vi "Configure Average.vi"(7 "Average On (F)":bool, 8 "error in (no error)":errorcluster, 10 "Average":u32, 11 "SA-ESA in":refnum<class "SA-ESA.lvclass">) -> (0 "error out":errorcluster, 3 "SA-ESA out":refnum<class "SA-ESA.lvclass">)   [LabVIEW 2020, in "SA-ESA.lvclass"]
uses:
  SA-ESA.lvclass
  C:/Sandbox/Git_Sandbox/WiSpry Test Framework source code (LV20)/WiSpry Test Framework/Instruments/Instrument.lvclass
  C:/Sandbox/Git_Sandbox/WiSpry Test Framework source code (LV20)/WiSpry Test Framework/Instruments/Spectrum Analyzer/Spectrum Analyzer.lvclass
  Spectrum Analyzer.lvclass/Spectrum Analyzer.ctl
  Instrument.lvclass/Instrument.ctl
  Instrument.lvclass
  Spectrum Analyzer.lvclass
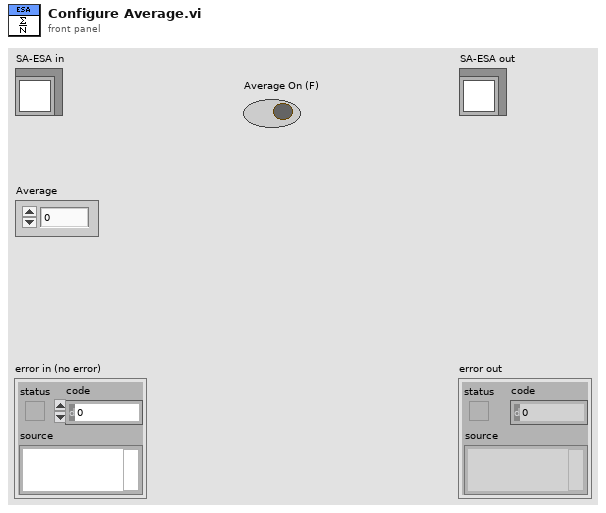
[diagram p1: front panel]
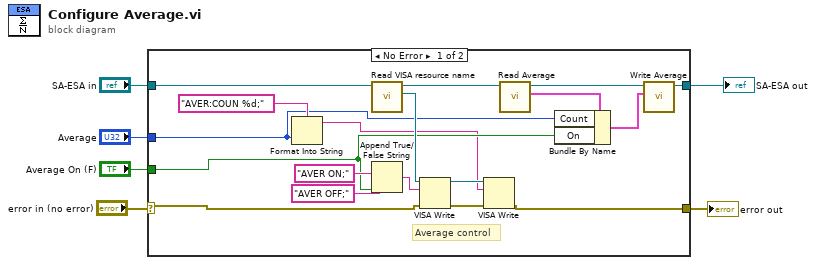
[diagram p0: block diagram]
diagram:
  n1 = case shown="No Error" "error in (no error)" {
    selector: "error in (no error)" -> [w18 w25]
    tunnel: "SA-ESA in" -> [w20 w26]
    tunnel: "Average" -> [w15 _]
    tunnel: "Average On (F)" -> [w14 _]
    tunnel: [w11 w26] -> w2
    tunnel: [w7 w25] -> w1
    frame No Error {
      # "Average control"
      n2 = Format Into String(format string="AVER:COUN %d;", w15) -> (resulting string=w8:string)  [unwired: 2 in, 1 out]
      n3 = call "Read VISA resource name.vi"("Instrument in"=w20) -> ("VISA resource name"=w19:refnum<visa-resource-name>, "Instrument out"=w17:refnum<class "SA-ESA.lvclass">)  [unwired: 9 in]
      n4 = Append True/False String(1:w14, 2:"AVER OFF;" ("false string"), 3:"AVER ON;" ("true string")) -> (0:w21:string)  [unwired: 1 in]
      n5 = VISA Write(VISA resource name=w19, write buffer=w21, error in (no error)=w18) -> (VISA resource name out=w9:refnum<visa-resource-name>, error out=w10:errorcluster)  [unwired: 1 out]
      n6 = VISA Write(VISA resource name=w9, write buffer=w8, error in (no error)=w10) -> (error out=w7:errorcluster)  [unwired: 2 out]
      n7 = call "Read Average.vi"("Spectrum Analyzer in"=w17) -> ("Average"=w16:cluster{"Count":u32, "On":bool}, "Spectrum Analyzer out"=w13:refnum<class "SA-ESA.lvclass">)  [unwired: 9 in]
      n8 = Bundle By Name(cluster=w16, "Count"=w15, "On"=w14) -> (w12:cluster{"Count":u32, "On":bool})
      n9 = call "Write Average.vi"("Average"=w12, "Spectrum Analyzer in"=w13) -> ("Spectrum Analyzer out"=w11:refnum<class "SA-ESA.lvclass">)  [unwired: 9 in]
    }
    frame Error {
    }
  }
  "error out" <- w1
  "SA-ESA out" <- w2
